vi "RSZVB Print Setup.vi"(0 "VISA session":refnum<visa-resource-name>, 1 "Diagram Area (0: All Diagram Areas)":i32(ring) items=["All Diagram Areas", "Active Diagram Area", "Single Diagram Area"], 2 "Logo (T: On)":bool=TRUE, 3 "Date and Time (T: On)":bool=TRUE, 4 "Marker List (T: On)":bool=TRUE, 5 "error in (no error)":errorcluster {"code" format="%.0x"}, 6 "Left Margin (0.01 mm)":dbl=0.01 format="%^.3e", 7 "Right Margin (0.01 mm)":dbl=0.01 format="%^.3e", 8 "Top Margin (0.01 mm)":dbl=0.01 format="%^.3e", 9 "Bottom Margin (0.01 mm)":dbl=0.01 format="%^.3e", 10 "Page Orientation (0: Portrait)":i32(ring) items=["Portrait", "Landscape"]) -> (14 "dup VISA session":refnum<visa-resource-name>, 19 "error out":errorcluster {"code" format="%.0x"})   [LabVIEW 2011]
doc: "This VI Provides options to specify how the document should be printed.\n\nNote(s):\n\nRemote-control command(s):\nHCOPy:ITEM:ALL\nHCOPy:ITEM:LOGO[:STATe] <Boolean>\nHCOPy:ITEM:MLISt[:STATe] <Boolean>\nHCOPy:ITEM:TIME[:STATe] <Boolean>\nHCOPy:PAGE:MARGin:LEFT <numeric_value>\nHCOPy:PAGE:MARGin:RIGHt <numeric_value>\nHCOPy:PAGE:MARGin:TOP <numeric_value>\nHCOPy:PAGE:MARGin:BOTTom <numeric_value>\nHCOPy:PAGE:ORIentation PORTrait | LANDscape\nHCOPy:PAGE:WINDow ALL | SINGle | ACTive"
panel:
  # "On\nOff"
  # "On\nOff"
  # "On\nOff"
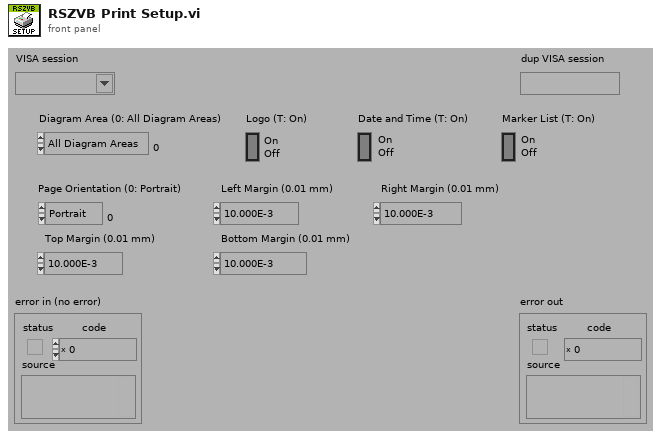
[diagram p1: front panel]
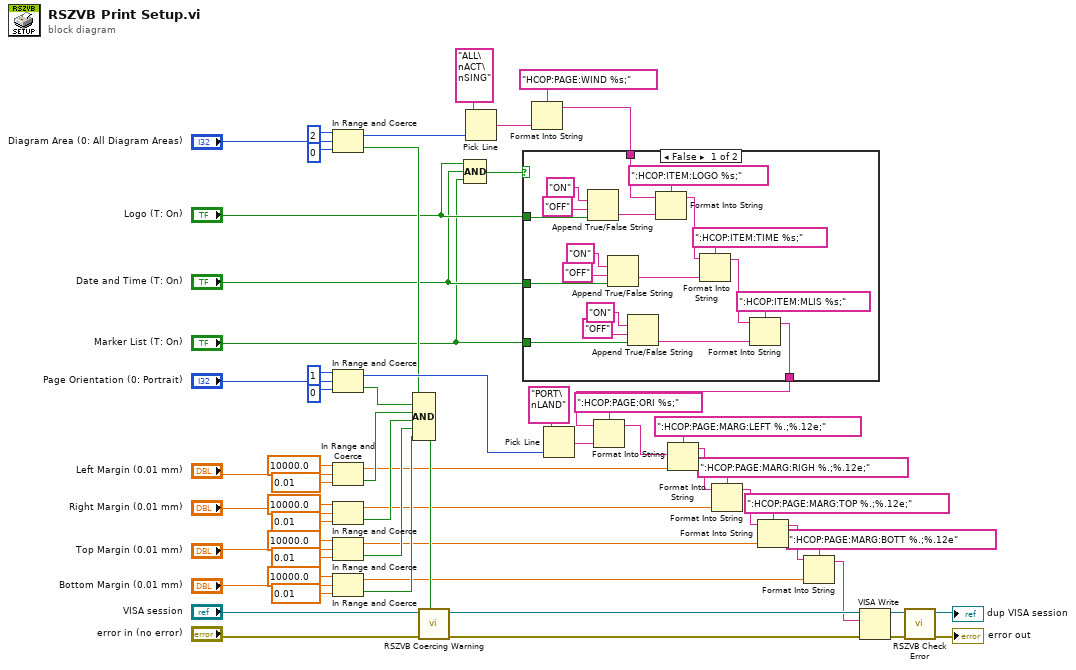
[diagram p0: block diagram]
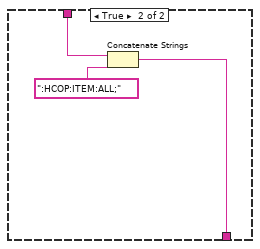
[diagram p2: hidden frame]
diagram:
  n1 = In Range and Coerce(upper limit=2, x="Diagram Area (0: All Diagram Areas)", lower limit=0) -> (coerced(x)=w46:i32, In Range?=w45:bool)
  n2 = In Range and Coerce(upper limit=1, x="Page Orientation (0: Portrait)", lower limit=0) -> (coerced(x)=w47:i32, In Range?=w44:bool)
  n3 = In Range and Coerce(upper limit=10000.0, x="Left Margin (0.01 mm)", lower limit=0.01) -> (coerced(x)=w10:dbl, In Range?=w18:bool)
  n4 = In Range and Coerce(upper limit=10000.0, x="Right Margin (0.01 mm)", lower limit=0.01) -> (coerced(x)=w9:dbl, In Range?=w17:bool)
  n5 = In Range and Coerce(upper limit=10000.0, x="Top Margin (0.01 mm)", lower limit=0.01) -> (coerced(x)=w8:dbl, In Range?=w16:bool)
  n6 = In Range and Coerce(upper limit=10000.0, x="Bottom Margin (0.01 mm)", lower limit=0.01) -> (coerced(x)=w7:dbl, In Range?=w15:bool)
  n7 = Compound Arithmetic op=AND(w45, w44, w18, w17, w16, w15) -> (w43:bool)
  n8 = call "RSZVB Coercing Warning.vi"("In Range?"=w43, "error in (no error)"="error in (no error)", "VISA session"="VISA session") -> ("error out"=w41:errorcluster, "dup VISA session"=w42:refnum<visa-resource-name>)  [unwired: 7 in]
  n9 = Compound Arithmetic op=AND("Logo (T: On)", "Date and Time (T: On)", "Marker List (T: On)") -> (w52:bool)
  n10 = Pick Line(multi-line string="ALL\nACT\nSING", line index=w46) -> (output string=w58:string)  [unwired: 1 in]
  n11 = Format Into String(format string="HCOP:PAGE:WIND %s;", w58) -> (resulting string=w31:string)  [unwired: 2 in, 1 out]
  n12 = case shown="False" w52 {
    tunnel: "Logo (T: On)" -> [w73 _]
    tunnel: "Date and Time (T: On)" -> [w72 _]
    tunnel: "Marker List (T: On)" -> [w71 _]
    tunnel: w31 -> [w62 w82]
    tunnel: [w61 w80] -> w1
    frame False {
      n13 = Append True/False String(1:w73, 2:"OFF", 3:"ON") -> (0:w67:string)  [unwired: 1 in]
      n14 = Append True/False String(1:w72, 2:"OFF", 3:"ON") -> (0:w66:string)  [unwired: 1 in]
      n15 = Append True/False String(1:w71, 2:"OFF", 3:"ON") -> (0:w65:string)  [unwired: 1 in]
      n16 = Format Into String(format string=":HCOP:ITEM:LOGO %s;", initial string=w62, w67) -> (resulting string=w64:string)  [unwired: 1 in, 1 out]
      n17 = Format Into String(format string=":HCOP:ITEM:TIME %s;", initial string=w64, w66) -> (resulting string=w63:string)  [unwired: 1 in, 1 out]
      n18 = Format Into String(format string=":HCOP:ITEM:MLIS %s;", initial string=w63, w65) -> (resulting string=w61:string)  [unwired: 1 in, 1 out]
    }
    frame True {
      n19 = Concatenate Strings(w82, ":HCOP:ITEM:ALL;") -> (w80:string)
    }
  }
  n20 = Pick Line(multi-line string="PORT\nLAND", line index=w47) -> (output string=w53:string)  [unwired: 1 in]
  n21 = Format Into String(format string=":HCOP:PAGE:ORI %s;", initial string=w1, w53) -> (resulting string=w6:string)  [unwired: 1 in, 1 out]
  n22 = Format Into String(format string=":HCOP:PAGE:MARG:LEFT %.;%.12e;", initial string=w6, w10) -> (resulting string=w5:string)  [unwired: 1 in, 1 out]
  n23 = Format Into String(format string=":HCOP:PAGE:MARG:RIGH %.;%.12e;", initial string=w5, w9) -> (resulting string=w4:string)  [unwired: 1 in, 1 out]
  n24 = Format Into String(format string=":HCOP:PAGE:MARG:TOP %.;%.12e;", initial string=w4, w8) -> (resulting string=w3:string)  [unwired: 1 in, 1 out]
  n25 = Format Into String(format string=":HCOP:PAGE:MARG:BOTT %.;%.12e", initial string=w3, w7) -> (resulting string=w2:string)  [unwired: 1 in, 1 out]
  n26 = VISA Write(VISA resource name=w42, write buffer=w2, error in (no error)=w41) -> (VISA resource name out=w60:refnum<visa-resource-name>, error out=w59:errorcluster)  [unwired: 1 out]
  n27 = call "RSZVB Check Error.vi"("error in (no error)"=w59, "VISA session"=w60) -> ("error out"=→"error out":errorcluster, "dup VISA session"=→"dup VISA session":refnum<visa-resource-name>)  [unwired: 8 in]
